vi "Temperature warning.vi"() -> ()   [LabVIEW 2022 SP3]
panel:
  out "Weather Data Out":T1
  in  "Weather Data In":T1
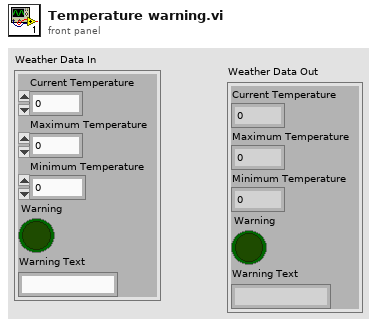
[diagram p1: front panel]
types:
  T1 = cluster{"Current Temperature":dbl, "Maximum Temperature":dbl, "Minimum Temperature":dbl, "Warning":bool, "Warning Text":string}
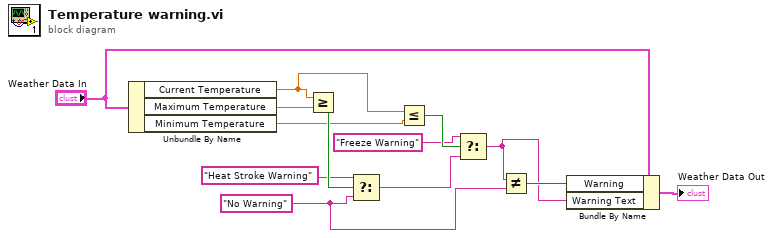
[diagram p0: block diagram]
diagram:
  w5 = "No Warning"
  n1 = Unbundle By Name("Weather Data In") -> ("Current Temperature"=w9:dbl, "Maximum Temperature"=w13:dbl, "Minimum Temperature"=w10:dbl)
  n2 = Greater Or Equal?(x=w9, y=w13) -> (x >= y?=w12:bool)
  n3 = Select(t="Heat Stroke Warning", s=w12, f=w5) -> (s? t:f=w6:string)
  n4 = Less Or Equal?(x=w9, y=w10) -> (x <= y?=w8:bool)
  n5 = Select(t="Freeze Warning", s=w8, f=w6) -> (s? t:f=w2:string)
  n6 = Not Equal?(x=w2, y=w5) -> (x != y?=w3:bool)
  n7 = Bundle By Name(cluster="Weather Data In", "Warning"=w3, "Warning Text"=w2) -> (→"Weather Data Out":T1)
